vi "Read Icon.vi"(8 "error in (no error)":errorcluster, 11 "TTLDevice in":refnum<class "TTLWaterDelivery.lvclass">) -> (0 "error out":errorcluster, 2 "Icon":picture, 3 "TTLDevice out":refnum<class "TTLWaterDelivery.lvclass">)   [LabVIEW 2020, in "TTLWaterDelivery.lvclass"]
uses:
  TTLWaterDelivery.lvclass
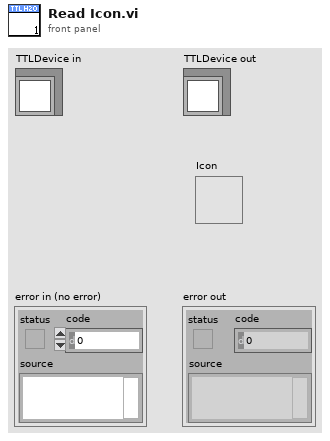
[diagram p1: front panel]
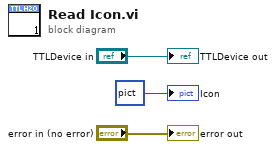
[diagram p0: block diagram]
diagram:
  "error out" <- "error in (no error)"
  "TTLDevice out" <- "TTLDevice in"
  "Icon" <- picture bytes[7230] ("Water")
